vi "readreference(sub).vi"(5 "element":refnum<vi>, 6 "errorin":errorcluster, 7 "appended array":refnum<vi>[](array[refnum]), 8 "Array":i32[](array[numeric])=[1, 2, 3, 4, 5, 1000, 1001, 1002, 1003, 0, 0], 9 "resourcein":refnum<visa-resource-name>) -> (0 "errorout 2":errorcluster, 1 "appended array 2":refnum<vi>[](array[refnum]), 2 "Array 2":i32[](array[numeric])=[1, 2, 3, 4, 5, 1000, 1001, 1002, 1003, 0, 0], 3 "resourceout":refnum<visa-resource-name>, 4 "readstring":string)   [LabVIEW 2015]
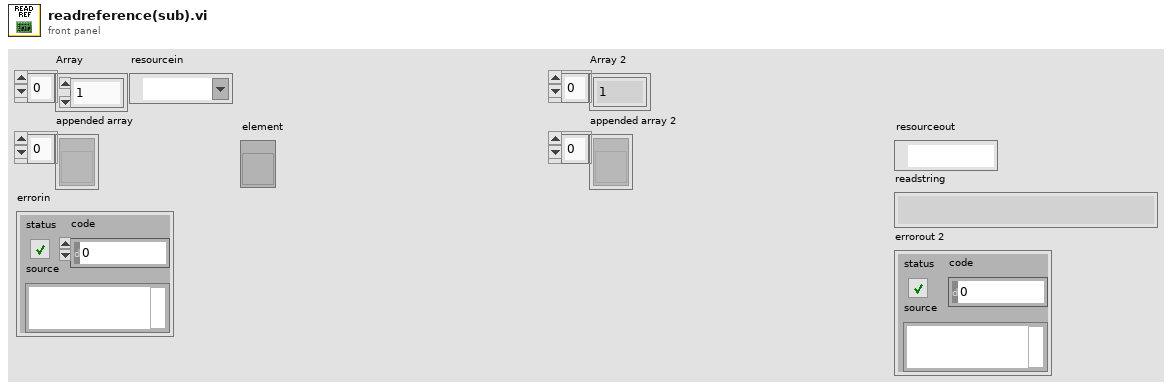
[diagram p1: front panel]
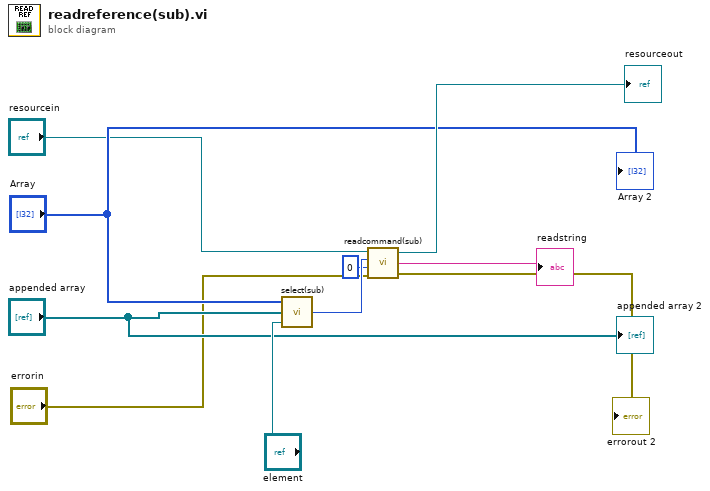
[diagram p0: block diagram]
diagram:
  n1 = call "select(sub).vi"("element"="element", "appended array"="appended array", "Array"="Array") -> ("command"=w10:i32)
  n2 = call "readcommand(sub).vi"("errorin"="errorin", "readdelay"=u32 0, "Command"=w10, "resourcein"="resourcein") -> ("errorout"=→"errorout 2":errorcluster, "readstring"=→"readstring":string, "resourceout"=→"resourceout":refnum<visa-resource-name>)
  "Array 2" <- "Array"
  "appended array 2" <- "appended array"
